vi "Command and response.vi"() -> ()   [LabVIEW 2017]
uses:
  Libraries/SSH/Response Configuration.ctl
  Libraries/SSH/Expected Response String Config.ctl
  Libraries/SSH/Search Start Point.ctl
  Libraries/SSH/Character Count Configuration.ctl
  Libraries/SSH/SSH.lvlib
panel:
  in  "Response Configuration":T1
  out "Response":string
  in  "Command":string
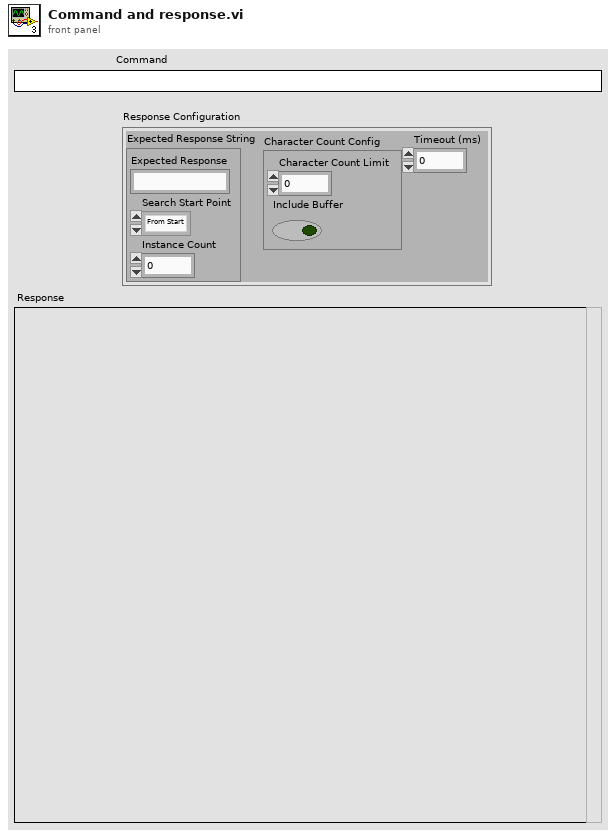
[diagram p1: front panel]
types:
  T1 = typedef "SSH.lvlib/Response Configuration.ctl" = cluster{"Expected Response String":T2, "Character Count Config":T4, "Timeout (ms)":i32}
  T2 = typedef "SSH.lvlib/Expected Response String Config.ctl" = cluster{"Expected Response":string, "Search Start Point":T3, "Instance Count":i32}
  T3 = typedef "SSH.lvlib/Search Start Point.ctl" = enum16{"From Start", "From End"}
  T4 = typedef "SSH.lvlib/Character Count Configuration.ctl" = cluster{"Character Count Limit":i32, "Include Buffer":bool}
  T5 = typedef "SSH.lvlib/Connection Info.ctl" = cluster{"host IP":string, "port":i32, "username":string, "password":string, "Connection Name":string}
  T6 = typedef "eventvkey.ctl" = enum16{"ASCII", "Enter", "Return", "Shift", "Ctrl", "Alt", "Cmd", "Opt", "Caps", "NumLock", "Clear", "Break", "Up", "Down", "Left", "Right", "Insert", "Delete", "Home", "End", "PageUp", "PageDown", "Escape", "Help", "Pause", "ScrollLock", "F1", "F2", "F3", "F4", "F5", "F6", "F7", "F8", "F9", "F10", "F11", "F12", "F13", "F14", "F15", "F16", "F17", "F18", "F19", "F20", "F21", "F22", "F23", "F24", "Play", "VolumeUp", "VolumeDown", "Mute", "Two Byte Char"}
  T7 = typedef "SSH.lvlib/Write Command (Reply Payload)--cluster.ctl" = cluster{"Write Command_error":errorcluster, "Return String Payload":string}
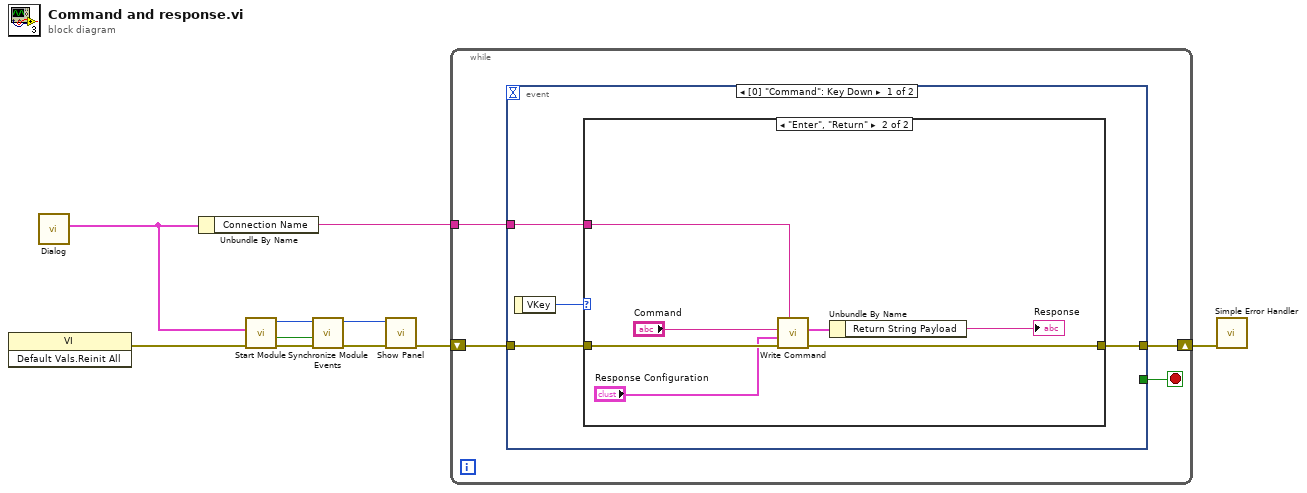
[diagram p0: block diagram]
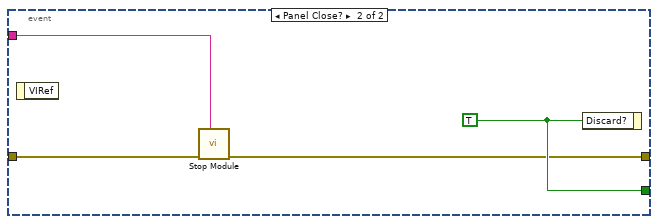
[diagram p3: hidden frame]
diagram:
  n1 = invoke class="VI" method="Default Vals.Reinit All"() -> (error out=w1:errorcluster)  [unwired: 3 in, 2 out]
  n2 = call "Dialog.vi"() -> ("Connection Info out"=w6:T5)  [unwired: 11 in]
  n3 = Unbundle By Name(w6) -> ("Connection Name"=w5:string)
  n4 = call "Start Module.vi"("error in (no error)"=w1, "Connection Info"=w6) -> ("error out"=w8:errorcluster, "Wait for Event Sync?"=w9:bool, "Module ID"=w10:i32)  [unwired: 6 in, 1 out]
  n5 = call "Synchronize Module Events.vi"("error in (no error)"=w8, "Wait for Event Sync?"=w9, "Module ID"=w10) -> ("error out"=w7:errorcluster, "Module ID (dup)"=w2:i32)  [unwired: 7 in]
  n6 = call "Show Panel.vi"("error in (no error)"=w7, "Module ID"=w2) -> ("error out"=w3:errorcluster)  [unwired: 9 in]
  n7 = while {
    tunnel: w5 -> [w13]
    shift-right: [w11] -> w4
    shift-left: w3 -> [w12]
    stop <- w14 stop-if-true
    n8 = event shown="[0] \"Command\": Key Down" {
      selector: _ -> [_ _]
      dyn-events: _ -> [_ _]
      timeout: _ -> [_ _]
      tunnel: [_ w30] -> w14
      tunnel: w13 -> [w18 w28]
      tunnel: w12 -> [w17 w29]
      tunnel: [w16 w27] -> w11
      event "Command": Key Down {
        n9 = event-data() -> ("VKey"=w15:T6)  [unwired: 1 in]
        n10 = case shown="\"Enter\", \"Return\"" w15 {
          tunnel: w18 -> [_ w26]
          tunnel: w17 -> [w19 w25]
          tunnel: [w19 w22] -> w16
          frame "ASCII", Default {
          }
          frame "Enter", "Return" {
            n11 = call "Write Command.vi"("Connection Name"=w26, "error in (no error)"=w25, "Response Configuration"="Response Configuration", "Command"="Command") -> ("error out"=w22:errorcluster, "Reply Payload"=w24:T7)  [unwired: 5 in, 1 out]
            n12 = Unbundle By Name(w24) -> ("Return String Payload"=→"Response":string)
          }
        }
      }
      event Panel Close? {
        w30 = TRUE ("Discard?")
        n13 = event-data() -> ()  [unwired: 1 in, 1 out]
        n14 = call "Stop Module.vi"("Connection Name"=w28, "error in (no error)"=w29) -> ("error out"=w27:errorcluster)  [unwired: 9 in]
        n15 = event-data("Discard?"=w30) -> ()  [unwired: 1 in, 1 out]
      }
    }
  }
  n16 = call <vilib>:"Simple Error Handler.vi"("error in (no error)"=w4) -> ()  [unwired: 4 in, 5 out]
